vi "Set Event Name.vi"(10 "Name (Generic)":string="Generic", 11 "Event In":refnum<class "Event.lvclass">) -> (3 "Event Out":refnum<class "Event.lvclass">)   [LabVIEW 2019, in "Event Source.lvlib" / "Event.lvclass"]
doc: "Set the name that will define the event. You can keep the input Event object unwired if you only specify the name for event. This can be used for example while unsubscribing i.e. when only the name is needed.\n\n<b>IMPORTANT</b> - If no name is wired or the wired string is empty, the name \"Generic\" will be set. This is to prevent errors with dictionary key name being empty."
uses:
  Event.lvclass
  Event.lvclass/Event.ctl
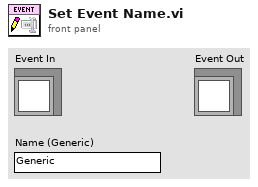
[diagram p1: front panel]
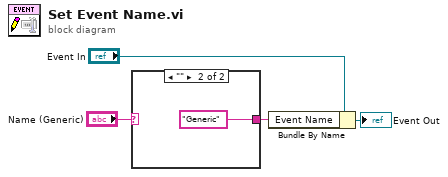
[diagram p0: block diagram]
diagram:
  n1 = case shown="\"\"" "Name (Generic)" {
    selector: "Name (Generic)" -> [w5 _]
    tunnel: [w5 "Generic"] -> w1
    frame Default {
    }
    frame "" {
    }
  }
  n2 = Bundle By Name(cluster="Event In", "Event Name"=w1) -> (→"Event Out":refnum<class "Event.lvclass">)
